vi "Read numOfInterleaves.vi"(8 "error in (no error)":errorcluster, 11 "BuckBoost configuration in":refnum<class "BuckBoost configuration.lvclass">) -> (0 "error out":errorcluster, 2 "numOfInterleaves":u8, 3 "BuckBoost configuration out":refnum<class "BuckBoost configuration.lvclass">)   [LabVIEW 2017, in "BuckBoost configuration.lvclass"]
uses:
  BuckBoost configuration.lvclass
  BuckBoost configuration.lvclass/BuckBoost configuration.ctl
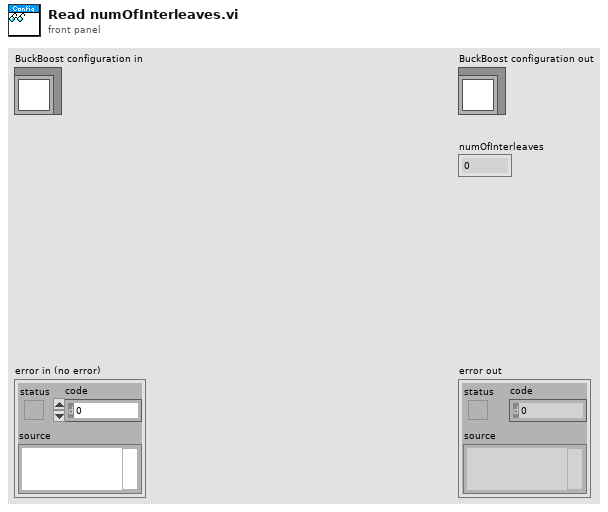
[diagram p1: front panel]
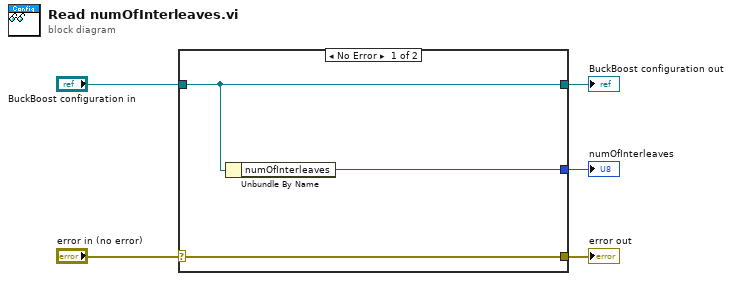
[diagram p0: block diagram]
diagram:
  n1 = case shown="No Error" "error in (no error)" {
    selector: "error in (no error)" -> [w8 w9]
    tunnel: [w8 w9] -> w4
    tunnel: [w7 w10] -> w2
    tunnel: "BuckBoost configuration in" -> [w7 w10]
    tunnel: [w6 _] -> w1
    frame No Error {
      n2 = Unbundle By Name(w7) -> ("numOfInterleaves"=w6:u8)
    }
    frame Error {
    }
  }
  "error out" <- w4
  "BuckBoost configuration out" <- w2
  "numOfInterleaves" <- w1
